vi "Test Driver.vi"() -> ()   [LabVIEW 2017]
uses:
  x64/Release/TestDriver States.ctl
  <vilib>/vision/Image Controls.llb/IMAQ Image.ctl
  x64/Release/BonTechWrapperLibrary.lvlib
panel:
  out "SendCapCommand Status":i32 format="%.0x"
  in  "Acquisition Mode":T1(ring)
  in  "Stop Continuous Acquisition":bool
  in  "Start Continuous  Acquisition":bool
  in  "Acquisition Commands (nMode)":u16(ring) items=["ACQ_INIT"=0, "DARK_MODE"=1, "BRIGHT_MODE"=2, "SOFTTRIGGER_MODE"=258, "SOFTTRIGGER_INSTANT_MODE"=259]
  out "Continous Acq function Status":i32 format="%.0x"
  out "nHeight out":u16
  out "nWidth out":u16
  in  "Error in (no error)":errorcluster
  in  "Disconnect":bool
  in  "Capture Image":bool
  in  "Configure":bool
  in  "Connect":bool
  out "Capture Status":i32 format="%.0x"
  out "Image":T2(plugin-control)
  in  "CalRefPath":string="C:\\\\BSD\\\\192.168.3.240\\\\Reference"
  in  "ConfigDir":string="C:\\\\BSD\\\\192.168.3.240\\\\Config"
  out "lpszSerialNum out":string
  out "Acq Mode Set Status":i32 format="%.0x"
  out "Error out":errorcluster
  out "Disconnect Status":i32 format="%.0x"
  out "Connect Status":i32 format="%.0x"
  in  "nSensorIP":string="192.168.3.240"
  in  "nHostIP":string="192.168.3.5"
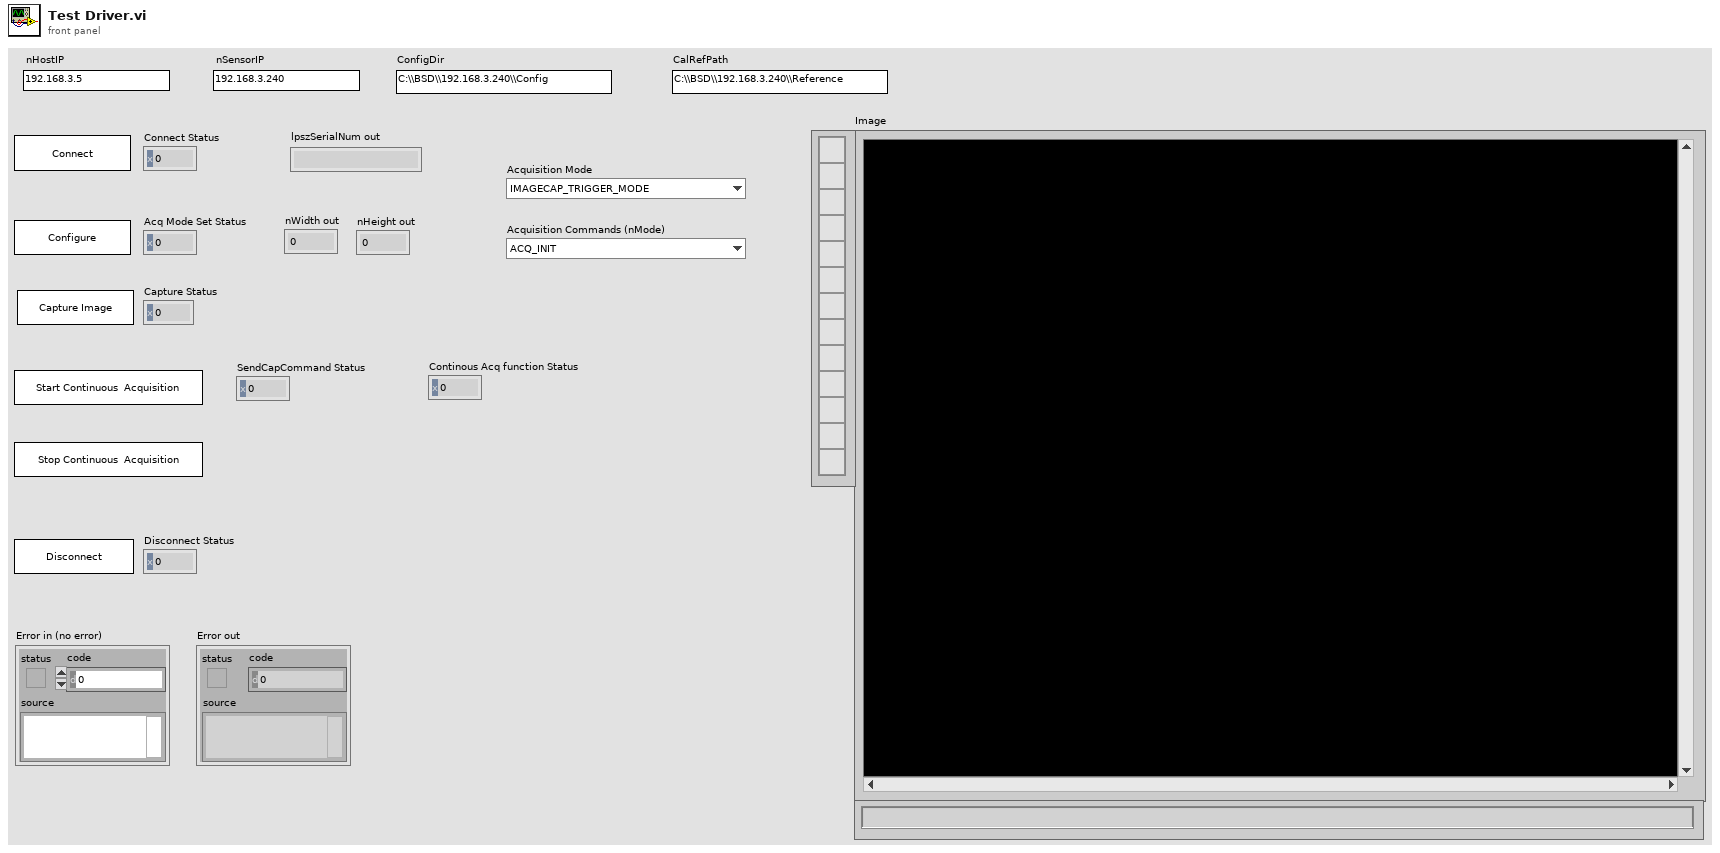
[diagram p1: front panel]
types:
  T1 = enum16{"IMAGECAP_TRIGGER_MODE", "IMAGECAP_AED_MODE", "IMAGECAP_SOFTTRIGGER_MODE", "IMAGECAP_AVG_COUNT_MODE", "IMAGECAP_AVG_AED_MODE", "IMAGECAP_CONTINUOUS_MODE", "IMAGECAP_CONTINUOUS_BINNING_MODE", "IMAGECAP_VIEWER_MODE"}
  T2 = typedef "IMAQ Image.ctl" = refnum<image>
  T3 = cluster{"nHostIP String":string, "nSensorIP String":string, "ConfigDir":string, "CalRefPath":string, "nMode":i32, "nAcqCommand":i32, "pImage":u16[], "ImageRef":T2, "nWidth":i32, "nHeight":i32, "nHostIP":u32, "nSensorIP":u32, "imgCapQ":refnum<queue>}
  T4 = typedef "TestDriver States.ctl" = enum16{"Poll", "Init", "Connect", "Configure", "Capture Image", "Disconnect", "Error", "Exit"}
  T5 = typedef "Image Type" = u32
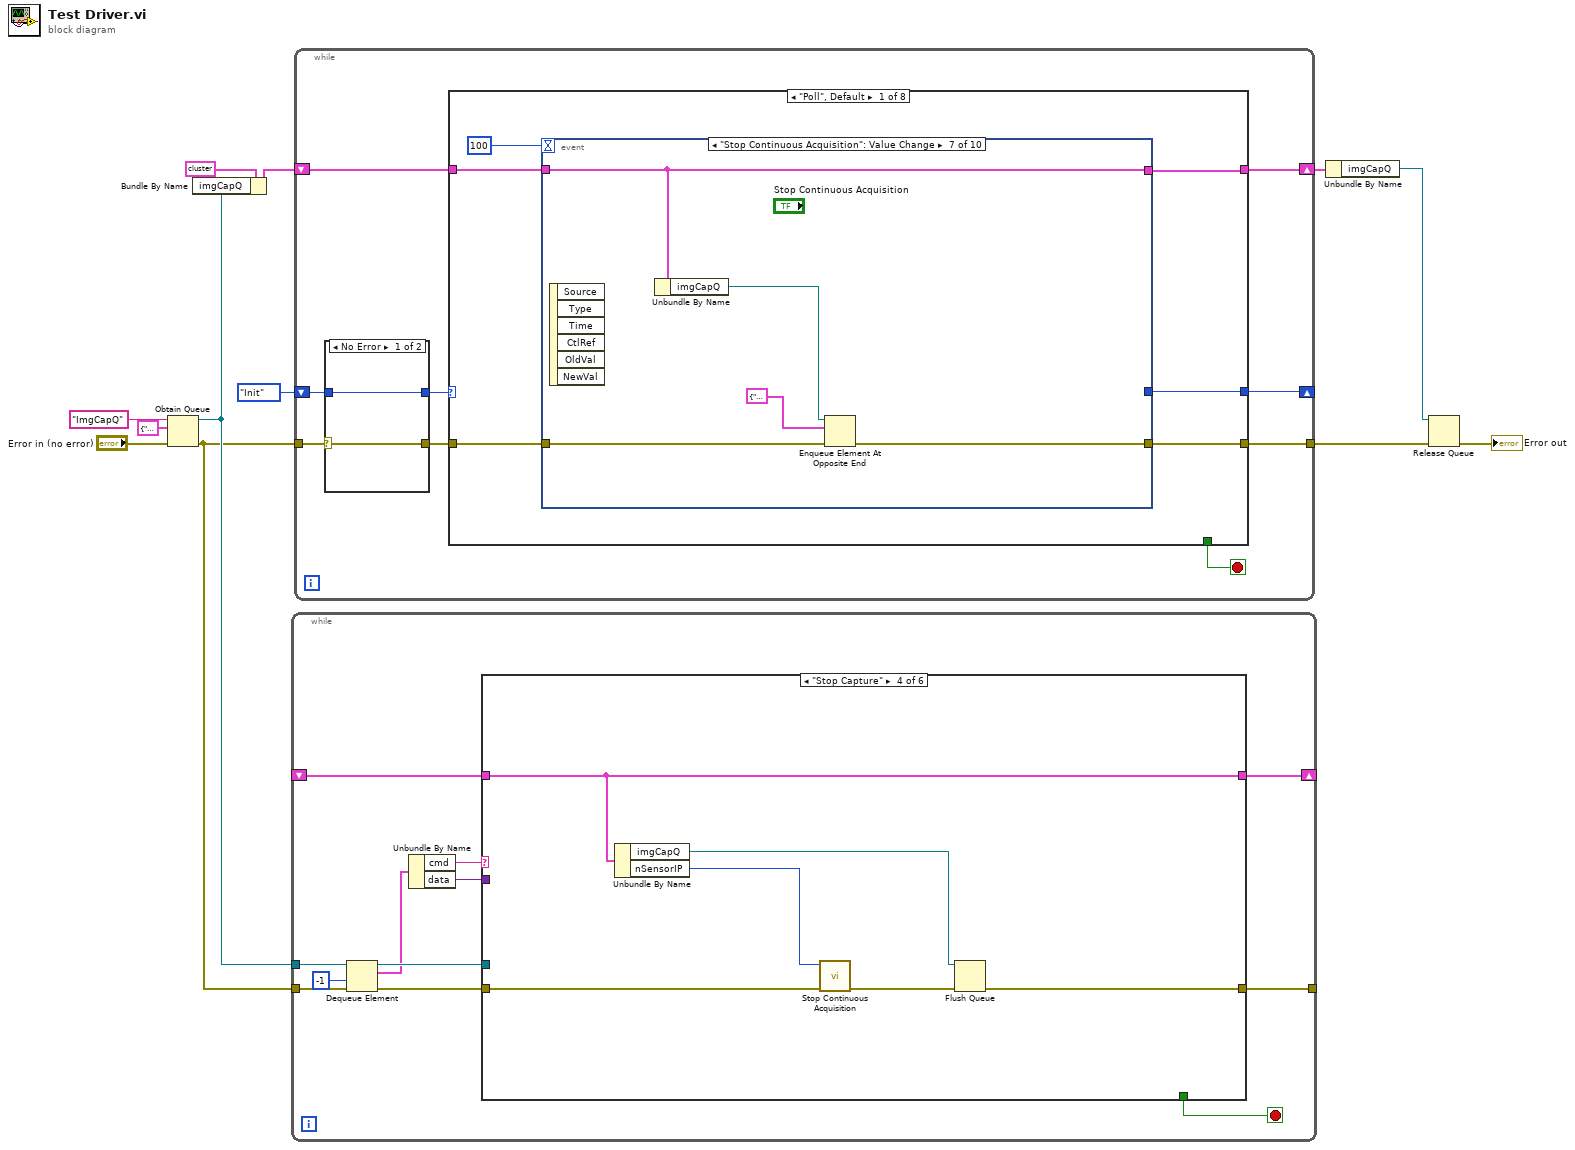
[diagram p0: block diagram]
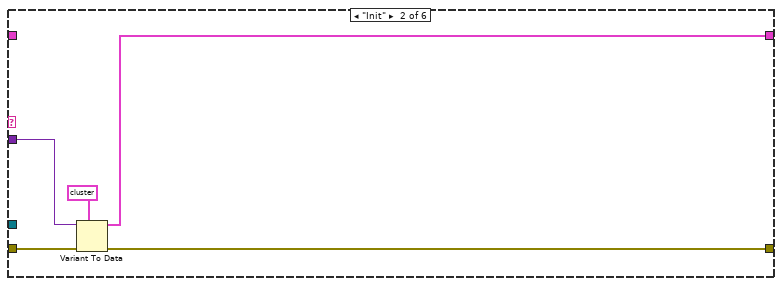
[diagram p3: hidden frame]
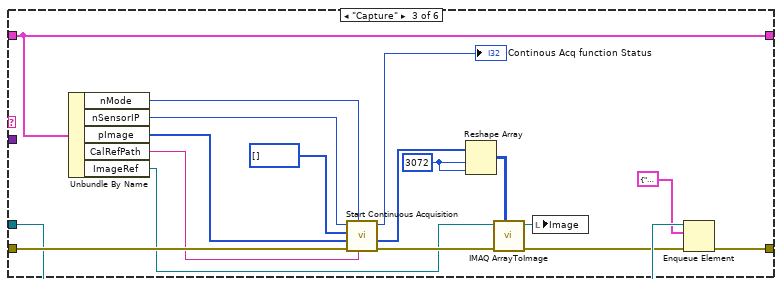
[diagram p4: hidden frame]
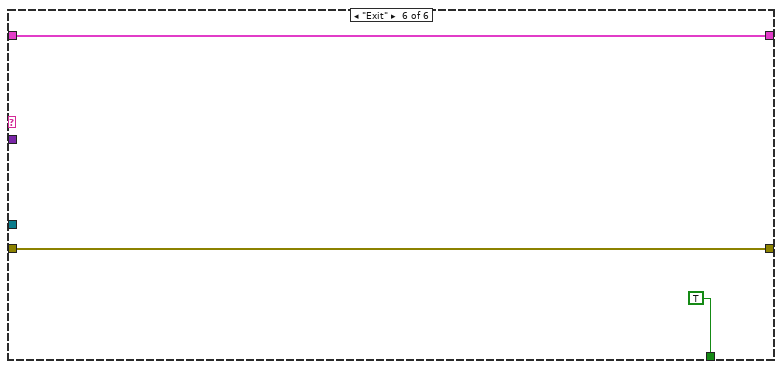
[diagram p6: hidden frame]
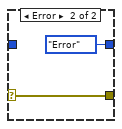
[diagram p7: hidden frame]
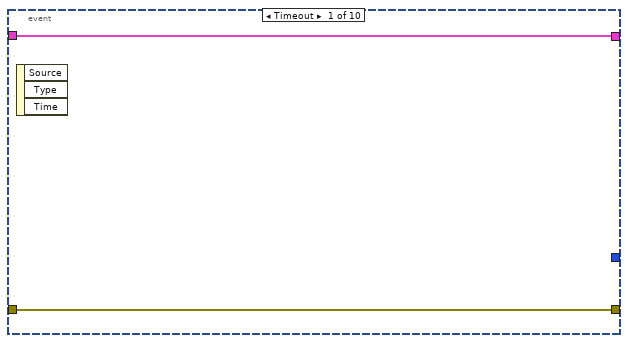
[diagram p8: hidden frame]
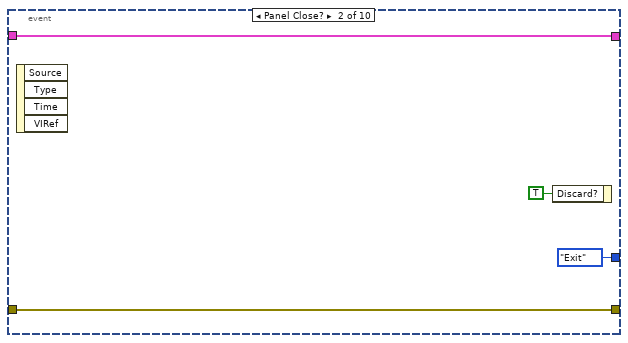
[diagram p9: hidden frame]
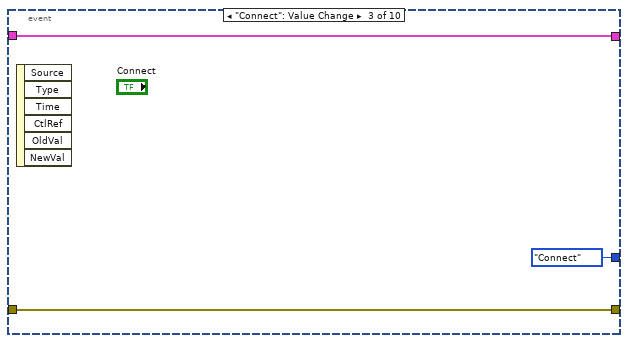
[diagram p10: hidden frame]
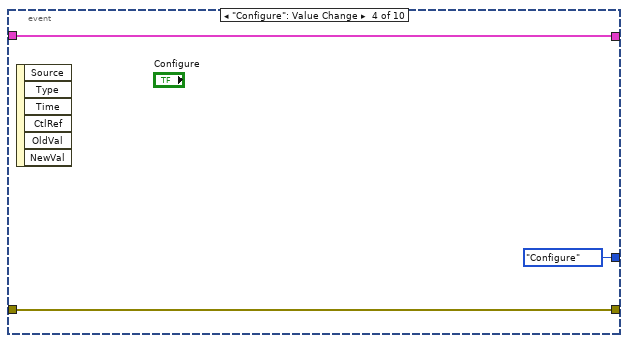
[diagram p11: hidden frame]
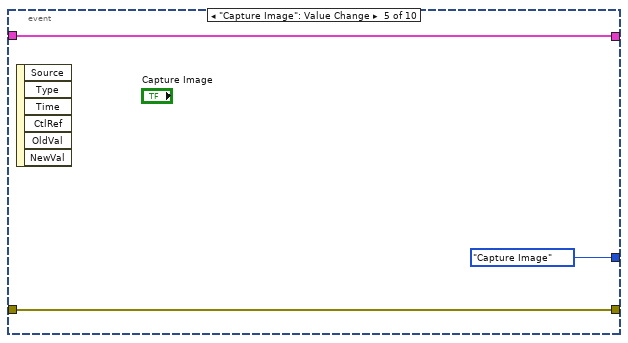
[diagram p12: hidden frame]
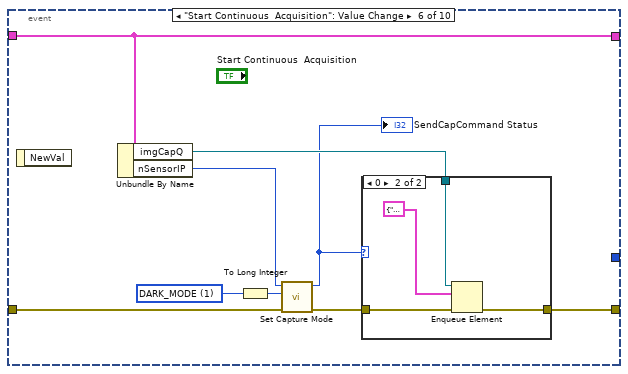
[diagram p13: hidden frame]
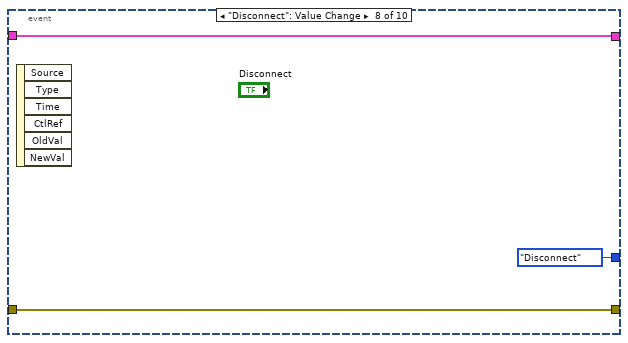
[diagram p15: hidden frame]
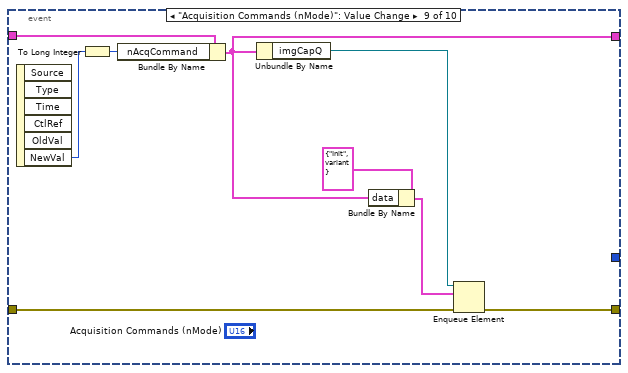
[diagram p16: hidden frame]
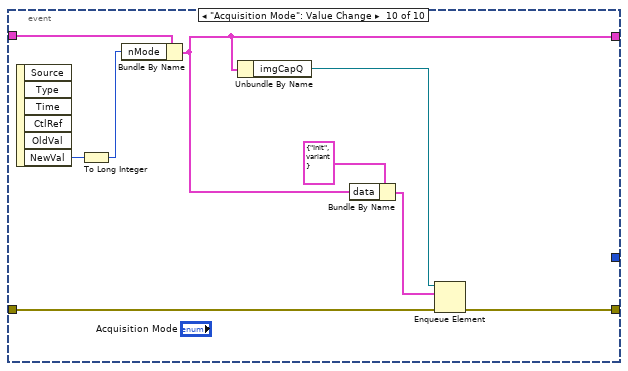
[diagram p17: hidden frame]
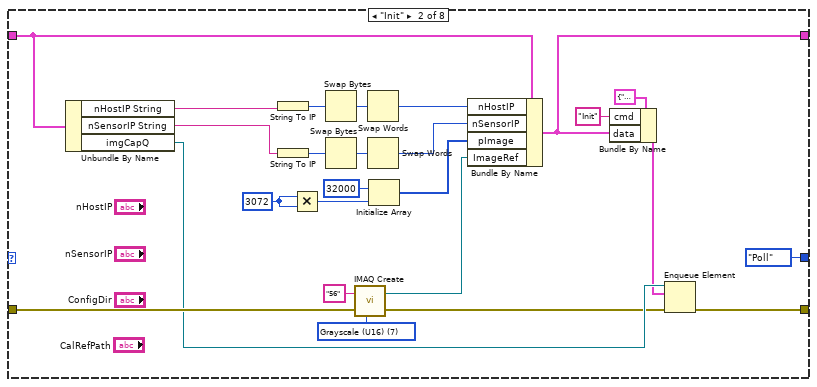
[diagram p18: hidden frame]
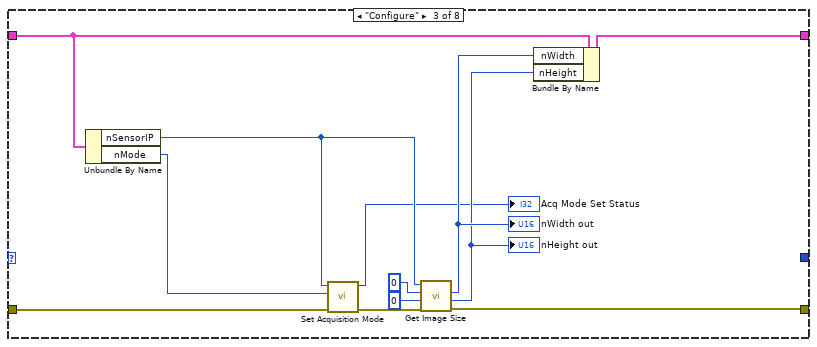
[diagram p19: hidden frame]
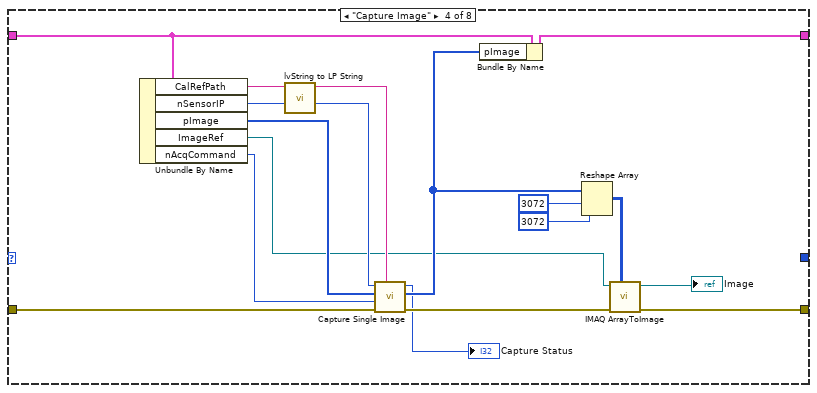
[diagram p20: hidden frame]
diagram:
  n1 = Obtain Queue(name (unnamed)="ImgCapQ", element data type=cluster{"cmd":string, "data":variant} {"cmd"="", "data"=variant}, error in (no error)="Error in (no error)") -> (queue out=w6:refnum<queue>, error out=w5:errorcluster)  [unwired: 2 in, 1 out]
  n2 = Bundle By Name(cluster=T3 {"nHostIP String"="192.168.3.5", "nSensorIP String"="192.168.3.240", "ConfigDir"="D:\\\\BSDx64\\\\192.168.3.240\\\\Config", "CalRefPath"="D:\\\\BSDx64\\\\192.168.3.240\\\\Reference", "nMode"=5, "nAcqCommand"=1, "pImage"=[], "ImageRef"=refnum, "nWidth"=3072, "nHeight"=3072, "nHostIP"=0, "nSensorIP"=0, "imgCapQ"=refnum}, "imgCapQ"=w6) -> (w7:T3)
  n3 = while {
    tunnel: w6 -> [w24]
    tunnel: w5 -> [w22]
    tunnel: [w19] -> _
    shift-right: [w14] -> _
    shift-left: _ -> [w13]
    stop <- w15 stop-if-true
    n4 = Dequeue Element(queue=w24, timeout in ms (-1)=-1, error in (no error)=w22) -> (queue out=w21:refnum<queue>, element=w18:cluster{"cmd":string, "data":variant}, error out=w20:errorcluster)  [unwired: 1 out]
    n5 = Unbundle By Name(w18) -> ("cmd"=w17:string, "data"=w16:variant)
    n6 = case shown="\"Stop Capture\"" w17 {
      tunnel: w21 -> [_ _ w37 _ _ _]
      tunnel: w20 -> [w26 w31 w49 w53 w56 w60]
      tunnel: [w26 w27 w35 w50 w56 w60] -> w19
      tunnel: w16 -> [_ w30 _ _ _ _]
      tunnel: [_ _ _ _ _ TRUE] -> w15
      tunnel: [w25 w28 w48 w55 w57 w58] -> w14
      tunnel: w13 -> [w25 _ w48 w55 w57 w58]
      frame "Idle", Default {
      }
      frame "Init" {
        n7 = Variant To Data(error in=w31, type=T3 {"nHostIP String"="192.168.3.5", "nSensorIP String"="192.168.3.240", "ConfigDir"="D:\\\\BSDx64\\\\192.168.3.240\\\\Config", "CalRefPath"="D:\\\\BSDx64\\\\192.168.3.240\\\\Reference", "nMode"=5, "nAcqCommand"=1, "pImage"=[], "ImageRef"=refnum, "nWidth"=3072, "nHeight"=3072, "nHostIP"=0, "nSensorIP"=0, "imgCapQ"=refnum}, Variant=w30) -> (data=w28:T3, error out=w27:errorcluster)
      }
      frame "Capture" {
        w33 = 3072 ("dimension size")
        n8 = Unbundle By Name(w48) -> ("nMode"=w32:i32, "nSensorIP"=w47:u32, "pImage"=w45:u16[], "CalRefPath"=w44:string, "ImageRef"=w38:T2)
        n9 = call "Start Continuous Acquisition.vi"("lpszRefPath"=w44, "nMode"=w32, "error in (no error)"=w49, "pImg"=w45, "refImg"=u16[] [], "nSensorIP"=w47) -> ("error out"=w43:errorcluster, "pImg out"=w41:u16[], "function return"=→"Continous Acq function Status":i32)  [unwired: 2 in, 1 out]
        n10 = Reshape Array(w41, w33, w33) -> (w42:u16[][])
        n11 = call "IMAQ ArrayToImage"("Image Pixels (U16)"=w42, "error in (no error)"=w43, "Image"=w38) -> ("error out"=w36:errorcluster, "Image Out"=w39:T2)  [unwired: 7 in]
        n12 = local write "Image"(w39) -> ()
        n13 = Enqueue Element(queue=w37, element=cluster{"cmd":string, "data":variant} {"cmd"="Capture", "data"=variant}, error in (no error)=w36) -> (error out=w35:errorcluster)  [unwired: 1 in, 2 out]
      }
      frame "Stop Capture" {
        n14 = Unbundle By Name(w55) -> ("imgCapQ"=w52:refnum<queue>, "nSensorIP"=w54:u32)
        n15 = call "Stop Continuous Acquisition.vi"("error in (no error)"=w53, "nSensorIP"=w54) -> ("error out"=w51:errorcluster)  [unwired: 8 in, 1 out]
        n16 = Flush Queue(queue=w52, error in (no error)=w51) -> (error out=w50:errorcluster)  [unwired: 2 out]
      }
      frame "Error" {
      }
      frame "Exit" {
      }
    }
  }
  n17 = while {
    shift-right: [w61] -> _
    shift-left: TestDriver_States."Init" -> [w65]
    tunnel: w5 -> [w69]
    shift-right: [w67] -> w2
    shift-left: w7 -> [w68]
    tunnel: [w63] -> w4
    stop <- w62 stop-if-true
    n18 = case shown="No Error" w69 {
      selector: w69 -> [w71 w73]
      tunnel: [w71 w73] -> w66
      tunnel: w65 -> [w70 _]
      tunnel: [w70 TestDriver_States."Error"] -> w64
      frame No Error {
      }
      frame Error {
      }
    }
    n19 = case shown="\"Poll\", Default" w64 {
      tunnel: w68 -> [w78 w156 w166 w187 w190 w195 w204 w214]
      tunnel: [w77 w136 w164 w182 w190 w195 w204 w214] -> w67
      tunnel: w66 -> [w76 w157 w168 w188 w189 w196 w206 w210]
      tunnel: [w75 w138 w167 w176 w189 w193 w205 w211] -> w63
      tunnel: [_ _ _ _ _ TRUE _ _] -> w62
      tunnel: [w74 TestDriver_States."Poll" _ _ _ _ _ TestDriver_States."Poll"] -> w61
      frame "Poll", Default {
        n20 = event shown="[6] \"Stop Continuous Acquisition\": Value Change" {
          selector: _ -> [_ _ _ _ _ _ _ _ _ _]
          dyn-events: _ -> [_ _ _ _ _ _ _ _ _ _]
          timeout: 100 -> [_ _ _ _ _ _ _ _ _ _]
          tunnel: [w81 w85 w88 w90 w94 w102 w111 w116 w118 w126] -> w77
          tunnel: w78 -> [w81 w85 w88 w90 w94 w102 w111 w116 w125 w127]
          tunnel: w76 -> [w80 w82 w86 w91 w93 w103 w113 w115 w121 w129]
          tunnel: [w80 w82 w86 w91 w93 w97 w112 w115 w120 w128] -> w75
          tunnel: [_ TestDriver_States."Exit" TestDriver_States."Connect" TestDriver_States."Configure" TestDriver_States."Capture Image" _ _ TestDriver_States."Disconnect" _ _] -> w74
          event Timeout {
            n21 = event-data() -> ()  [unwired: 1 in, 3 out]
          }
          event Panel Close? {
            n22 = event-data() -> ()  [unwired: 1 in, 4 out]
            n23 = event-data("Discard?"=TRUE) -> ()  [unwired: 1 in, 1 out]
          }
          event "Connect": Value Change {
            n24 = event-data() -> ()  [unwired: 1 in, 6 out]
          }
          event "Configure": Value Change {
            n25 = event-data() -> ()  [unwired: 1 in, 6 out]
          }
          event "Capture Image": Value Change {
            n26 = event-data() -> ()  [unwired: 1 in, 6 out]
          }
          event "Start Continuous  Acquisition": Value Change {
            w100 = u16 1 items=["ACQ_INIT"=0, "DARK_MODE"=1, "BRIGHT_MODE"=2, "SOFTTRIGGER_MODE"=258, "SOFTTRIGGER_INSTANT_MODE"=259] ("Acquisition Commands (nMode)")
            n27 = event-data() -> ()  [unwired: 1 in, 1 out]
            n28 = Unbundle By Name(w102) -> ("imgCapQ"=w96:refnum<queue>, "nSensorIP"=w101:u32)
            n29 = To Long Integer(number=w100) -> (32bit integer=w99:i32)
            n30 = call "Set Capture Mode.vi"("error in (no error)"=w103, "nMode"=w99, "nSensorIP"=w101) -> ("error out"=w98:errorcluster, "function return"=w95:i32)  [unwired: 7 in]
            "SendCapCommand Status" <- w95
            n31 = case shown="0" w95 {
              tunnel: w98 -> [w104 w108]
              tunnel: [w104 w107] -> w97
              tunnel: w96 -> [_ w106]
              frame 1, Default {
              }
              frame 0 {
                n32 = Enqueue Element(queue=w106, element=cluster{"cmd":string, "data":variant} {"cmd"="Capture", "data"=variant}, error in (no error)=w108) -> (error out=w107:errorcluster)  [unwired: 1 in, 2 out]
              }
            }
          }
          event "Stop Continuous Acquisition": Value Change {
            n33 = event-data() -> ()  [unwired: 1 in, 6 out]
            n34 = Unbundle By Name(w111) -> ("imgCapQ"=w110:refnum<queue>)
            n35 = Enqueue Element At Opposite End(queue=w110, element=cluster{"cmd":string, "data":variant} {"cmd"="Stop Capture", "data"=variant}, error in (no error)=w113) -> (error out=w112:errorcluster)  [unwired: 1 in, 2 out]
          }
          event "Disconnect": Value Change {
            n36 = event-data() -> ()  [unwired: 1 in, 6 out]
          }
          event "Acquisition Commands (nMode)": Value Change {
            n37 = event-data() -> ("NewVal"=w124:u16)  [unwired: 1 in, 5 out]
            n38 = To Long Integer(number=w124) -> (32bit integer=w123:i32)
            n39 = Bundle By Name(cluster=w125, "nAcqCommand"=w123) -> (w118:T3)
            n40 = Unbundle By Name(w118) -> ("imgCapQ"=w117:refnum<queue>)
            n41 = Bundle By Name(cluster=cluster{"cmd":string, "data":variant} {"cmd"="Init", "data"=variant} ("element"), "data"=w118) -> (w119:cluster{"cmd":string, "data":variant})
            n42 = Enqueue Element(queue=w117, element=w119, error in (no error)=w121) -> (error out=w120:errorcluster)  [unwired: 1 in, 2 out]
          }
          event "Acquisition Mode": Value Change {
            n43 = event-data() -> ("NewVal"=w134:T1)  [unwired: 1 in, 5 out]
            n44 = To Long Integer(number=w134) -> (32bit integer=w133:i32)
            n45 = Bundle By Name(cluster=w127, "nMode"=w133) -> (w126:T3)
            n46 = Unbundle By Name(w126) -> ("imgCapQ"=w131:refnum<queue>)
            n47 = Bundle By Name(cluster=cluster{"cmd":string, "data":variant} {"cmd"="Init", "data"=variant} ("element"), "data"=w126) -> (w132:cluster{"cmd":string, "data":variant})
            n48 = Enqueue Element(queue=w131, element=w132, error in (no error)=w129) -> (error out=w128:errorcluster)  [unwired: 1 in, 2 out]
          }
        }
      }
      frame "Init" {
        w143 = 3072 ("x")
        w158 = T5 7 items=["Grayscale (U8)", "Grayscale (I16)", "Grayscale (SGL)", "Complex (CSG)", "RGB (U32)", "HSL (U32)", "RGB (U64)", "Grayscale (U16)"] ("Image Type")
        n49 = Unbundle By Name(w156) -> ("nHostIP String"=w151:string, "nSensorIP String"=w150:string, "imgCapQ"=w141:refnum<queue>)
        n50 = String To IP(1:w151) -> (0:w154:u32)
        n51 = String To IP(1:w150) -> (0:w155:u32)
        n52 = Multiply(x=w143, y=w143) -> (x*y=w147:i32)
        n53 = Swap Bytes(anything=w154) -> (byte swapped=w153:u32)
        n54 = Swap Bytes(anything=w155) -> (byte swapped=w152:u32)
        n55 = call "IMAQ Create"("Image Name"="56", "Image Type"=w158, "error in (no error)"=w157) -> ("New Image"=w145:T2, "error out"=w139:errorcluster)  [unwired: 2 in]
        n56 = Swap Words(1:w153) -> (0:w148:u32)
        n57 = Swap Words(1:w152) -> (0:w149:u32)
        n58 = Initialize Array(u16 32000, w147) -> (w144:u16[])
        n59 = Bundle By Name(cluster=w156, "nHostIP"=w148, "nSensorIP"=w149, "pImage"=w144, "ImageRef"=w145) -> (w136:T3)
        n60 = Bundle By Name(cluster=cluster{"cmd":string, "data":variant} {"cmd"="", "data"=variant} ("element"), "cmd"="Init", "data"=w136) -> (w137:cluster{"cmd":string, "data":variant})
        n61 = Enqueue Element(queue=w141, element=w137, error in (no error)=w139) -> (error out=w138:errorcluster)  [unwired: 1 in, 2 out]
      }
      frame "Configure" {
        n62 = Unbundle By Name(w166) -> ("nSensorIP"=w165:u32, "nMode"=w160:i32)
        n63 = call "Set Acquisition Mode.vi"("error in (no error)"=w168, "nMode"=w160, "nSensorIP"=w165) -> ("error out"=w171:errorcluster, "function return"=→"Acq Mode Set Status":i32)  [unwired: 7 in]
        n64 = call "Get Image Size.vi"("error in (no error)"=w171, "nHeight"=u16 0, "nWidth"=u16 0, "nSensorIP"=w165) -> ("error out"=w167:errorcluster, "nHeight out"=w162:u16, "nWidth out"=w163:u16)  [unwired: 4 in, 1 out]
        "nWidth out" <- w163
        "nHeight out" <- w162
        n65 = Bundle By Name(cluster=w166, "nWidth"=w163, "nHeight"=w162) -> (w164:T3)
      }
      frame "Capture Image" {
        n66 = Unbundle By Name(w187) -> ("CalRefPath"=w185:string, "nSensorIP"=w186:u32, "pImage"=w183:u16[], "ImageRef"=w174:T2, "nAcqCommand"=w172:i32)
        n67 = call "lvString to LP String.vi"("LVString"=w185) -> ("LPTSTR String"=w184:string)  [unwired: 10 in]
        n68 = call "Capture Single Image.vi"("calRefPath"=w184, "error in (no error)"=w188, "nMode"=w172, "pImage"=w183, "nSensorIP"=w186) -> ("error out"=w177:errorcluster, "pImage out"=w178:u16[], "function return"=→"Capture Status":i32)  [unwired: 4 in]
        n69 = Bundle By Name(cluster=w187, "pImage"=w178) -> (w182:T3)
        n70 = Reshape Array(w178, 3072 ("dimension size"), 3072 ("dimension size")) -> (w179:u16[][])
        n71 = call "IMAQ ArrayToImage"("Image Pixels (U16)"=w179, "error in (no error)"=w177, "Image"=w174) -> ("error out"=w176:errorcluster, "Image Out"=→"Image":T2)  [unwired: 7 in]
      }
      frame "Error" {
      }
      frame "Exit" {
        n72 = Unbundle By Name(w195) -> ("imgCapQ"=w192:refnum<queue>, "ImageRef"=w194:T2)
        n73 = call "IMAQ Dispose"("Image"=w194, "error in (no error)"=w196) -> ("error out"=w193:errorcluster)  [unwired: 4 in]
        n74 = invoke class="VI" method="Default Vals.Reinit All"() -> ()  [unwired: 3 in, 3 out]
        n75 = Enqueue Element(queue=w192, element=cluster{"cmd":string, "data":variant} {"cmd"="Exit", "data"=variant}) -> ()  [unwired: 2 in, 3 out]
      }
      frame "Connect" {
        n76 = Unbundle By Name(w204) -> ("nHostIP"=w203:u32, "nSensorIP"=w200:u32, "ConfigDir"=w202:string)
        n77 = call "lvString to LP String.vi"("LVString"=w202) -> ("LPTSTR String"=w201:string)  [unwired: 10 in]
        n78 = call "Connect.vi"("error in (no error)"=w206, "ConfigDir"=w201, "nSensorIP"=w200, "nHostIP"=w203) -> ("error out"=w207:errorcluster, "function return"=→"Connect Status":i32)  [unwired: 5 in, 1 out]
        n79 = call "Get Serial Number.vi"("error in (no error)"=w207, "nSensorIP"=w200) -> ("error out"=w205:errorcluster, "lpszSerialNum out"=→"lpszSerialNum out":string)  [unwired: 7 in, 1 out]
      }
      frame "Disconnect" {
        n80 = Unbundle By Name(w214) -> ("nSensorIP"=w208:u32)
        n81 = call "Cancel Single Image Capture.vi"("error in (no error)"=w210, "nSensorIP"=w208) -> ("error out"=w209:errorcluster)  [unwired: 8 in, 1 out]
        n82 = call "Disconnect.vi"("error in (no error)"=w209, "nSensorIP"=w208) -> ("error out"=w211:errorcluster, "function return"=→"Disconnect Status":i32)  [unwired: 8 in]
        n83 = invoke class="VI" method="Default Vals.Reinit All"(error in=w211) -> ()  [unwired: 2 in, 3 out]
      }
    }
  }
  n84 = Unbundle By Name(w2) -> ("imgCapQ"=w1:refnum<queue>)
  n85 = Release Queue(queue=w1, error in (no error)=w4) -> (error out=→"Error out":errorcluster)  [unwired: 1 in, 2 out]
